vi "StateGripper.vi"(0 "Master State In":T1(ring)) -> ()   [LabVIEW 2020]
doc: "This VI makes all decisions related to the gripper subsystem."
uses:
  GlobalDriverStationCommands.vi
  GlobalGripper.vi
  GlobalArm.vi
  GlobalPoseAndTargeting.vi
panel:
  in  "Cube Hold Power":dbl=0.06
  in  "Cone Hold Power":dbl=0.04
  in  "Cube Outtake Power":dbl=-1.0
  in  "Cone Outtake Power":dbl=-1.0
  in  "Cone Intake Power":dbl=0.7
  in  "Cube Intake Power":dbl=1.0
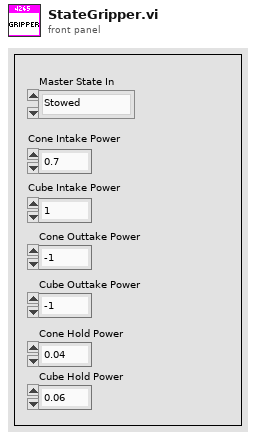
[diagram p1: front panel]
types:
  T1 = enum16{"Stowed", "Balancing", "Scoring", "Hoppering", "Ground", "Shelf"}
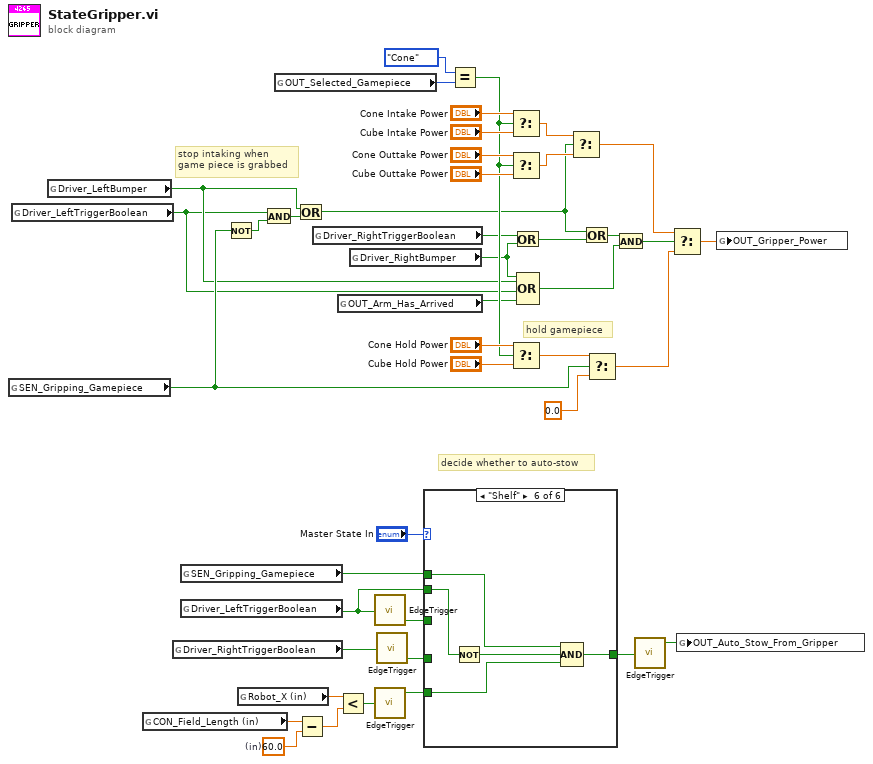
[diagram p0: block diagram]
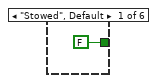
[diagram p2: hidden frame]
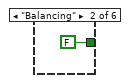
[diagram p3: hidden frame]
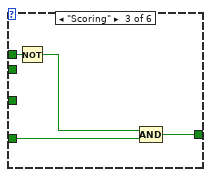
[diagram p4: hidden frame]
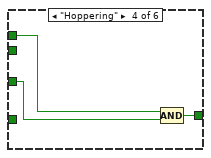
[diagram p5: hidden frame]
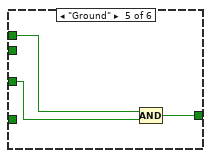
[diagram p6: hidden frame]
diagram:
  w4 = 60.0  # (in)
  # "decide whether to auto-stow"
  # "stop intaking when\ngame piece is grabbed"
  # "hold gamepiece"
  n1 = global read "GlobalGripper.vi" "SEN_Gripping_Gamepiece"() -> (w23:bool)
  n2 = global read "GlobalDriverStationCommands.vi" "Driver_LeftTriggerBoolean"() -> (w1:bool)
  n3 = global read "GlobalDriverStationCommands.vi" "Driver_LeftBumper"() -> (w10:bool)
  n4 = global read "GlobalPoseAndTargeting.vi" "CON_Field_Length (in)"() -> (w5:dbl)
  n5 = global read "GlobalDriverStationCommands.vi" "Driver_RightTriggerBoolean"() -> (w22:bool)
  n6 = global read "GlobalGripper.vi" "SEN_Gripping_Gamepiece"() -> (w19:bool)
  n7 = global read "GlobalDriverStationCommands.vi" "Driver_LeftTriggerBoolean"() -> (w6:bool)
  n8 = Not(x=w23) -> (.not. x?=w24:bool)
  n9 = global read "GlobalPoseAndTargeting.vi" "Robot_X (in)"() -> (w9:dbl)
  n10 = And(x=w1, y=w24) -> (x .and. y?=w16:bool)
  n11 = global read "GlobalArm.vi" "OUT_Selected_Gamepiece"() -> (w37:enum16{"Cube", "Cone"})
  n12 = Or(x=w10, y=w16) -> (x .or. y?=w15:bool)
  n13 = Subtract(x=w5, y=w4) -> (x-y=w3:dbl)
  n14 = global read "GlobalDriverStationCommands.vi" "Driver_RightTriggerBoolean"() -> (w12:bool)
  n15 = global read "GlobalArm.vi" "OUT_Arm_Has_Arrived"() -> (w2:bool)
  n16 = Less?(x=w9, y=w3) -> (x < y?=w8:bool)
  n17 = global read "GlobalDriverStationCommands.vi" "Driver_RightBumper"() -> (w11:bool)
  n18 = call "EdgeTrigger.vi"("Input Signal"=w6) -> ("Falling Edge Trigger"=w20:bool)  [unwired: 2 out]
  n19 = call "EdgeTrigger.vi"("Input Signal"=w8) -> ("Rising Edge Trigger"=w7:bool)  [unwired: 2 out]
  n20 = call "EdgeTrigger.vi"("Input Signal"=w22) -> ("Falling Edge Trigger"=w21:bool)  [unwired: 2 out]
  n21 = case shown="\"Shelf\"" "Master State In" {
    tunnel: [FALSE FALSE w49 w52 w55 w59] -> w18
    tunnel: w21 -> [_ _ w48 _ _ _]
    tunnel: w19 -> [_ _ w47 w50 w53 w56]
    tunnel: w20 -> [_ _ _ w51 w54 _]
    tunnel: w7 -> [_ _ _ _ _ w60]
    tunnel: w6 -> [_ _ _ _ _ w58]
    frame "Stowed", Default {
    }
    frame "Balancing" {
    }
    frame "Scoring" {
      n22 = Not(x=w47) -> (.not. x?=w46:bool)
      n23 = Compound Arithmetic op=AND(w46, w48) -> (w49:bool)
    }
    frame "Hoppering" {
      n24 = Compound Arithmetic op=AND(w50, w51) -> (w52:bool)
    }
    frame "Ground" {
      n25 = Compound Arithmetic op=AND(w53, w54) -> (w55:bool)
    }
    frame "Shelf" {
      n26 = Not(x=w58) -> (.not. x?=w57:bool)
      n27 = Compound Arithmetic op=AND(w56, w57, w60) -> (w59:bool)
    }
  }
  n28 = Equal?(x=enum16{"Cube", "Cone"}."Cone", y=w37) -> (x = y?=w25:bool)
  n29 = Select(t="Cone Intake Power", s=w25, f="Cube Intake Power") -> (s? t:f=w27:dbl)
  n30 = Select(t="Cone Outtake Power", s=w25, f="Cube Outtake Power") -> (s? t:f=w26:dbl)
  n31 = Select(t="Cone Hold Power", s=w25, f="Cube Hold Power") -> (s? t:f=w30:dbl)
  n32 = Or(x=w12, y=w11) -> (x .or. y?=w14:bool)
  n33 = Compound Arithmetic op=OR(w11, w10, w1, w2) -> (w13:bool)
  n34 = Select(t=w27, s=w15, f=w26) -> (s? t:f=w31:dbl)
  n35 = Or(x=w15, y=w14) -> (x .or. y?=w34:bool)
  n36 = Select(t=w30, s=w23, f=0.0) -> (s? t:f=w28:dbl)
  n37 = And(x=w34, y=w13) -> (x .and. y?=w32:bool)
  n38 = call "EdgeTrigger.vi"("Input Signal"=w18) -> ("Rising Edge Trigger"=w17:bool)  [unwired: 2 out]
  n39 = Select(t=w31, s=w32, f=w28) -> (s? t:f=w33:dbl)
  n40 = global write "GlobalGripper.vi" "OUT_Auto_Stow_From_Gripper"(w17) -> ()
  n41 = global write "GlobalGripper.vi" "OUT_Gripper_Power"(w33) -> ()
